vi "Database Folder.vi"(3 "Relative Path (\"\" - Folder)":string) -> (1 "Data Folder":path)   [LabVIEW 2011]
uses:
  Spartan CONFIG Global.vi
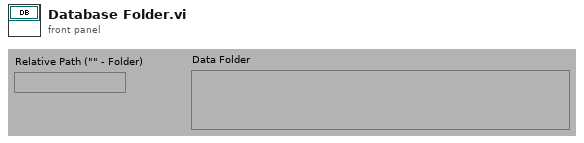
[diagram p1: front panel]
types:
  T1 = typedef "Keyed Array.ctl" = cluster{"keys":string[], "values":string[]}
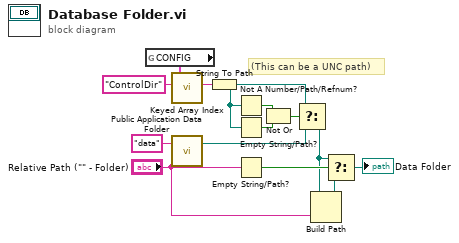
[diagram p0: block diagram]
diagram:
  # "(This can be a UNC path)"
  n1 = global read "Spartan CONFIG Global.vi" "CONFIG"() -> (w5:T1)
  n2 = call "Keyed Array Index.vi"("key"="ControlDir" ("name or relative path"), "array in"=w5) -> ("value"=w3:string)  [unwired: 2 in, 3 out]
  n3 = call "Public Application Data Folder.vi"("Relative Path (\"\" - Folder)"="data" ("name or relative path")) -> ("Client Storage Path"=w1:path)  [unwired: 2 in]
  n4 = String To Path(string=w3) -> (path=w6:path)
  n5 = Not A Number/Path/Refnum?(number/path/refnum=w6) -> (NaN/Path/Refnum?=w8:bool)
  n6 = Empty String/Path?(string/path=w6) -> (empty?=w9:bool)
  n7 = Empty String/Path?(string/path="Relative Path (\"\" - Folder)") -> (empty?=w13:bool)
  n8 = Not Or(1:w9, 2:w8) -> (0:w7:bool)
  n9 = Select(t=w6, s=w7, f=w1) -> (s? t:f=w10:path)
  n10 = Build Path(base path=w10, name or relative path="Relative Path (\"\" - Folder)") -> (appended path=w11:path)
  n11 = Select(t=w10, s=w13, f=w11) -> (s? t:f=→"Data Folder":path)
